vi "get img by id.vi"(8 "error in (no error)":errorcluster, 10 "id":i32, 11 "Test in":refnum<class "Test.lvclass">) -> (0 "error out":errorcluster, 3 "Test out":refnum<class "Test.lvclass">)   [LabVIEW 2013, in "DatenKlassen.lvlib" / "Test.lvclass"]
uses:
  Test.lvclass
  Test.lvclass/Test.ctl
  Image/img.lvclass
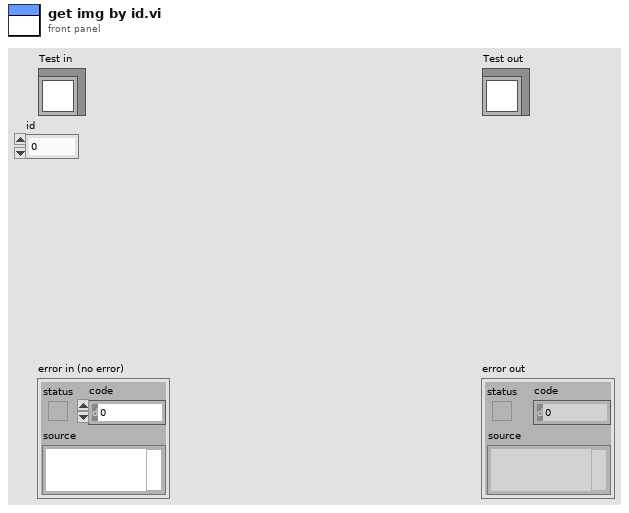
[diagram p1: front panel]
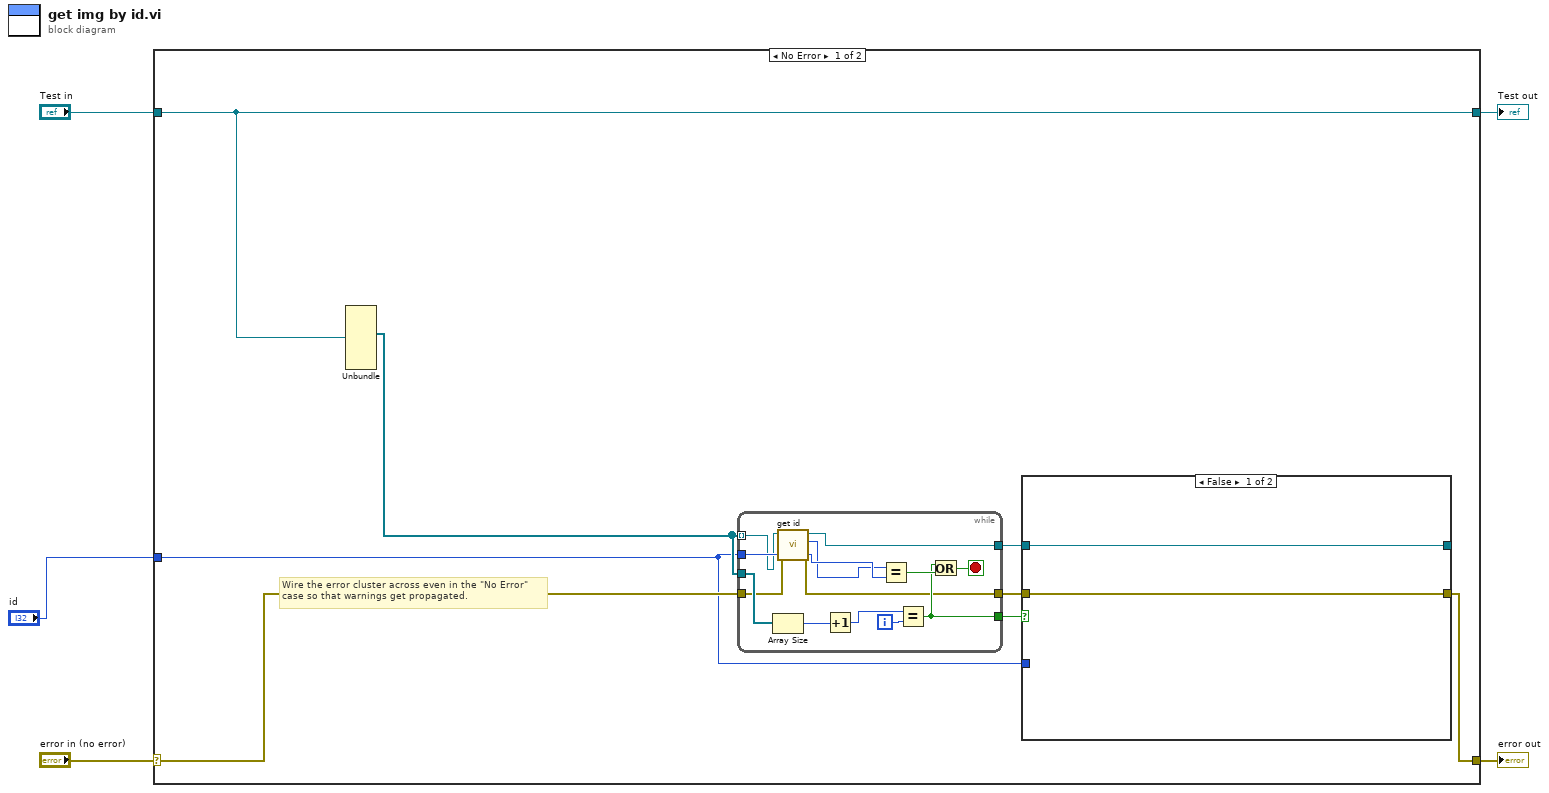
[diagram p0: block diagram]
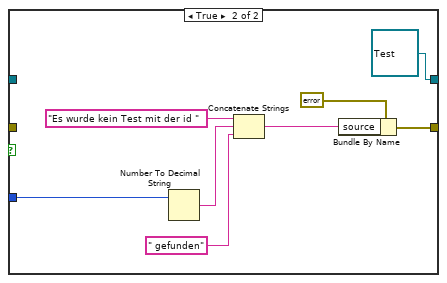
[diagram p2: hidden frame]
diagram:
  n1 = case shown="No Error" "error in (no error)" {
    selector: "error in (no error)" -> [w10 w38]
    tunnel: [w9 w38] -> w4
    tunnel: [w8 w37] -> w2
    tunnel: "Test in" -> [w8 w37]
    tunnel: "id" -> [w6 _]
    frame No Error {
      # "Wire the error cluster across even in the \"No Error\"\ncase so that warnings get propagated."
      n2 = Unbundle(w8) -> (w7:refnum<class "img.lvclass">[])  [unwired: 7 out]
      n3 = while {
        tunnel: w7 -> [w28] mode=indexing
        tunnel: w10 -> [w27]
        tunnel: w6 -> [w36]
        tunnel: [w26] -> w12
        tunnel: w7 -> [w35]
        tunnel: [w29] -> w11
        tunnel: [w25] -> w13
        i -> [w34]
        stop <- w32 stop-if-true
        n4 = Array Size(array=w35) -> (size(s)=w31:i32)
        n5 = call-dynamic "get id.vi"("error in (no error)"=w27, "img in"=w28) -> ("error out"=w26:errorcluster, "id"=w24:i32, "img out"=w25:refnum<class "img.lvclass">)  [unwired: 7 in]
        n6 = Increment(x=w31) -> (x+1=w30:i32)
        n7 = Equal?(x=w24, y=w36) -> (x = y?=w33:bool)
        n8 = Equal?(x=w30, y=w34) -> (x = y?=w29:bool)
        n9 = Or(x=w29, y=w33) -> (x .or. y?=w32:bool)
      }
      n10 = case shown="False" w11 {
        tunnel: w12 -> [w14 _]
        tunnel: w6 -> [_ w21]
        tunnel: [w14 w18] -> w9
        tunnel: [w15 refnum<class "Test.lvclass"> refnum ("Test out")] -> _
        tunnel: w13 -> [w15 _]
        frame False {
        }
        frame True {
          n11 = Number To Decimal String(number=w21) -> (decimal integer string=w20:string)  [unwired: 1 in]
          n12 = Concatenate Strings("Es wurde kein Test mit der id " ("source"), w20, " gefunden" ("string")) -> (w17:string)
          n13 = Bundle By Name(cluster=errorcluster {"status"=TRUE, "code"=9999, "source"="Es wurde kein Test mit der id "} ("error constant"), "source"=w17) -> (w18:errorcluster)
        }
      }
    }
    frame Error {
    }
  }
  "error out" <- w4
  "Test out" <- w2
